vi "Finish.vi"(8 "error in (no error)":errorcluster, 11 "Comp Motors with Encoders in":refnum<class "Comp Motors with Encoders.lvclass">) -> (0 "error out":errorcluster, 3 "Comp Motors with Encoders out":refnum<class "Comp Motors with Encoders.lvclass">)   [LabVIEW 2014, in "Comp Motors with Encoders.lvlib" / "Comp Motors with Encoders.lvclass"]
uses:
  Comp Motors with Encoders.lvclass
  Comp Motors with Encoders.lvclass/Comp Motors with Encoders.ctl
  Robot/Motor with Encoders/Motors with Encoders Class/Motors with Encoders.lvclass
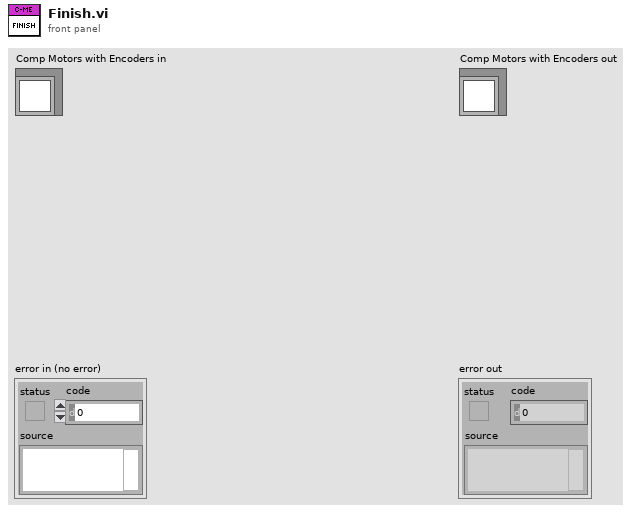
[diagram p1: front panel]
types:
  T1 = typedef "WPI_MotorControlDeviceRef.ctl" = cluster{"DeviceStatus":errorcluster, "Type":T2, "PWM":cluster{"Controller":T3, "PWM Channel":T4, "DeadBand":T5}, "CAN":cluster{"Device Number":u8, "Control Mode":T6, "Semaphore":T7, "Max Vout":dbl, "TalonSRX Control Mode":T8}, "Invert":bool, "TransformRef":T9, "InvTransformRef":T9}
  T2 = typedef "WPI_MotorControlType.ctl" = enum16{"PWM", "CAN", "CANTalonSRX"}
  T3 = typedef "FPGA_TypedefDigitalModule.ctl" = enum16{"Controller 1"}
  T4 = typedef "FPGA_DIOPWMChannel.ctl" = enum8{"PWM 0", "PWM 1", "PWM 2", "PWM 3", "PWM 4", "PWM 5", "PWM 6", "PWM 7", "PWM 8", "PWM 9", "PWM MXP 0", "PWM MXP 1", "PWM MXP 2", "PWM MXP 3", "PWM MXP 4", "PWM MXP 5", "PWM MXP 6", "PWM MXP 7", "PWM MXP 8", "PWM MXP 9", "Invalid"}
  T5 = typedef "WPI_PWMDeadband.ctl" = cluster{"Name":string, "maxPositivePwm":i32, "minPositivePwm":i32, "centerPwm":i32, "maxNegativePwm":i32, "minNegativePwm":i32, "angularRange":u16}
  T6 = typedef "WPI_CANJaguar_ControlMode.ctl" = enum8{"Percent VBus", "Current", "Speed", "Position", "Voltage"}
  T7 = typedef "Semaphore RefNum" = refnum<k1>
  T8 = typedef "WPI_CANTalonSRX_APIControlMode.ctl" = enum8{"Percent VBus", "Speed", "Position", "Slave", "Unchanged / Invalid"}
  T9 = typedef "WPI_PWMTransform_ConPane.ctl" = refnum<vi>
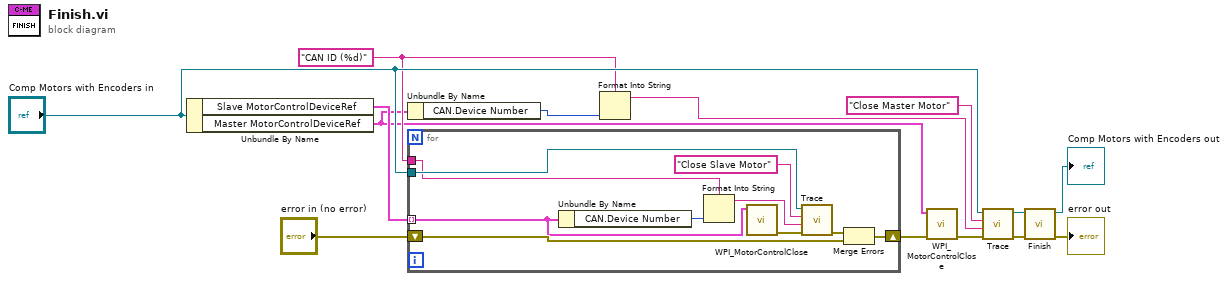
[diagram p0: block diagram]
diagram:
  w5 = "CAN ID (%d)" ("format string")
  n1 = Unbundle By Name("Comp Motors with Encoders in") -> ("Slave MotorControlDeviceRef"=w12:T1[], "Master MotorControlDeviceRef"=w4:T1)
  n2 = Unbundle By Name(w4) -> ("CAN.Device Number"=w3:u8)
  n3 = for {
    tunnel: w12 -> [w18] mode=indexing
    shift-right: [w20] -> w10
    shift-left: "error in (no error)" -> [w24]
    tunnel: "Comp Motors with Encoders in" -> [w23]
    tunnel: w5 -> [w15]
    n4 = Unbundle By Name(w18) -> ("CAN.Device Number"=w17:u8)
    n5 = Format Into String(format string=w15, w17) -> (resulting string=w16:string)  [unwired: 2 in, 1 out]
    n6 = call <vilib>:"WPI_MotorControlClose.vi"("MotorControlDevRef"=w18) -> ("error out"=w21:errorcluster)  [unwired: 10 in]
    n7 = call-dynamic "Trace.vi"("error in (no error)"=w21, "System Message"=w16, "System Action"="Close Slave Motor", "System Actor in"=w23) -> ("error out"=w19:errorcluster)  [unwired: 6 in, 1 out]
    n8 = Merge Errors(w19, w24) -> (w20:errorcluster)
  }
  n9 = Format Into String(format string=w5, w3) -> (resulting string=w2:string)  [unwired: 2 in, 1 out]
  n10 = call <vilib>:"WPI_MotorControlClose.vi"("error in (no error)"=w10, "MotorControlDevRef"=w4) -> ("error out"=w9:errorcluster)  [unwired: 9 in]
  n11 = call-dynamic "Trace.vi"("error in (no error)"=w9, "System Message"=w2, "System Action"="Close Master Motor", "System Actor in"="Comp Motors with Encoders in") -> ("error out"=w1:errorcluster, "System Actor out"=w7:refnum<class "Comp Motors with Encoders.lvclass">)  [unwired: 6 in]
  n12 = call-parent "Finish.vi"("error in (no error)"=w1, "System Actor in"=w7) -> ("error out"=→"error out":errorcluster, "System Actor out"=→"Comp Motors with Encoders out":refnum<class "Comp Motors with Encoders.lvclass">)  [unwired: 8 in]
